vi "read_params.vi"(8 "error in (no error)":errorcluster, 11 "TheilSenRegressor in":refnum<class "TheilSenRegressor.lvclass">) -> (0 "error out":errorcluster, 2 "params":T1={"fit_intercept"=TRUE, "copy_X"=TRUE, "max_subpopulation"=10000.0, "n_subsamples"={"n_subsamples_type"="None", "n_subsamples_int"=0.0}, "max_iter"=300.0, "tol"=0.001, "random_state"=0.0, "n_jobs"=1.0, "verbose"=FALSE}, 3 "TheilSenRegressor out":refnum<class "TheilSenRegressor.lvclass">)   [LabVIEW 2020, in "TheilSenRegressor.lvclass"]
uses:
  TheilSenRegressor.lvclass
  Controls/theilsen_regressor_params.ctl
  TheilSenRegressor.lvclass/TheilSenRegressor.ctl
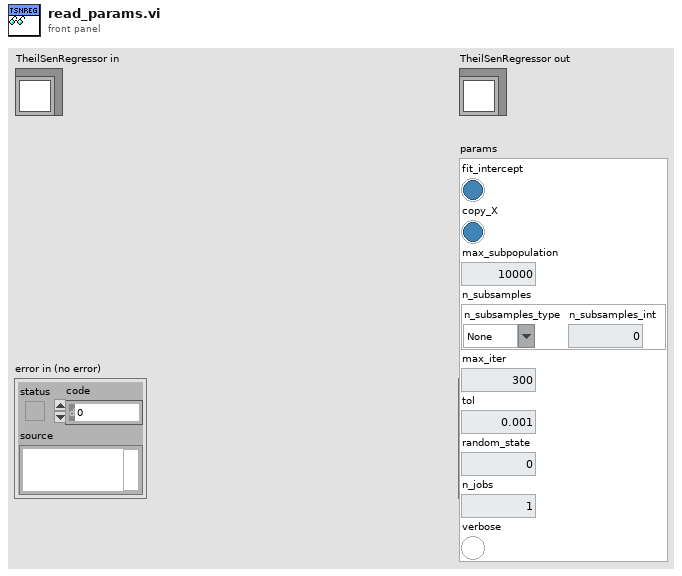
[diagram p1: front panel]
types:
  T1 = typedef "theilsen_regressor_params.ctl" = cluster{"fit_intercept":bool, "copy_X":bool, "max_subpopulation":dbl, "n_subsamples":cluster{"n_subsamples_type":string, "n_subsamples_int":dbl}, "max_iter":dbl, "tol":dbl, "random_state":dbl, "n_jobs":dbl, "verbose":bool}
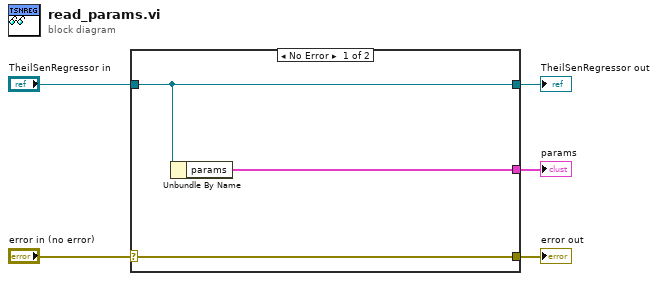
[diagram p0: block diagram]
diagram:
  n1 = case shown="No Error" "error in (no error)" {
    selector: "error in (no error)" -> [w8 w9]
    tunnel: [w8 w9] -> w4
    tunnel: [w7 w10] -> w2
    tunnel: "TheilSenRegressor in" -> [w7 w10]
    tunnel: [w6 _] -> w1
    frame No Error {
      n2 = Unbundle By Name(w7) -> ("params"=w6:T1)
    }
    frame Error {
    }
  }
  "error out" <- w4
  "TheilSenRegressor out" <- w2
  "params" <- w1
